vi "A_weighting_calculation.vi"(11 "Frequency":dbl) -> (2 "A(f)":dbl, 3 "Ra(f)":dbl)   [LabVIEW 2020]
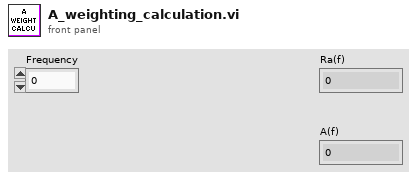
[diagram p1: front panel]
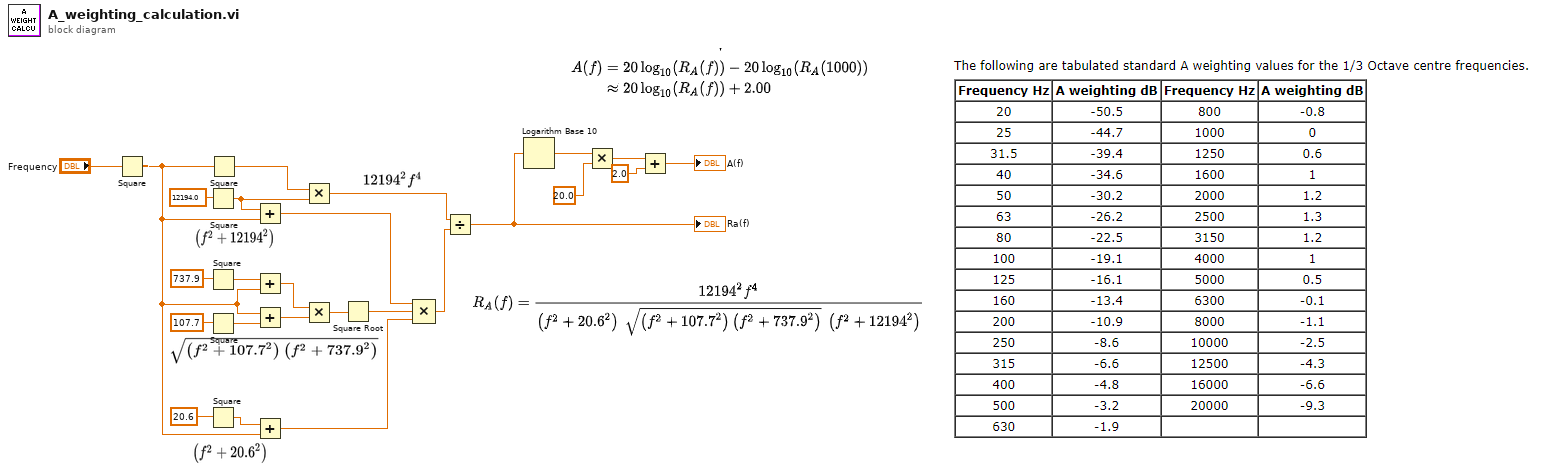
[diagram p0: block diagram]
diagram:
  n1 = Square(x="Frequency") -> (x^2=w5:dbl)
  n2 = Square(x=12194.0) -> (x^2=w4:dbl)
  n3 = Square(x=737.9) -> (x^2=w18:dbl)
  n4 = Square(x=107.7) -> (x^2=w19:dbl)
  n5 = Square(x=20.6) -> (x^2=w23:dbl)
  n6 = Square(x=w5) -> (x^2=w13:dbl)
  n7 = Add(x=w4, y=w5) -> (x+y=w2:dbl)
  n8 = Add(x=w18, y=w5) -> (x+y=w17:dbl)
  n9 = Add(x=w5, y=w19) -> (x+y=w16:dbl)
  n10 = Add(x=w23, y=w5) -> (x+y=w3:dbl)
  n11 = Multiply(x=w13, y=w4) -> (x*y=w12:dbl)
  n12 = Multiply(x=w17, y=w16) -> (x*y=w15:dbl)
  n13 = Square Root(x=w15) -> (sqrt(x)=w14:dbl)
  n14 = Compound Arithmetic op=MULTIPLY(w2, w14, w3) -> (w11:dbl)
  n15 = Divide(x=w12, y=w11) -> (x/y=w9:dbl)
  "Ra(f)" <- w9
  n16 = Logarithm Base 10(1:w9) -> (0:w8:dbl)
  n17 = Multiply(x=w8, y=20.0) -> (x*y=w7:dbl)
  n18 = Add(x=w7, y=2.0) -> (x+y=→"A(f)":dbl)
